vi "Main.vi"(8 "init information":string, 9 "model name":string, 11 "Module Admin":refnum<class "Delacor_lib_QMH_Cloneable Module Admin.lvclass">) -> ()   [LabVIEW 2022 SP3, in "Model Thread.lvlib"]
doc: "This template is based off of the Queued Message Handler design pattern and the Queued Message Handler project template that ships with LabVIEW.\n\nThe main difference is that the queue is private to this module and communication between modules is performed via Broadcast and Request events.\n\nRequest events are wrapped in public API methods and are handled in the Event Handling Loop (EHL) of this VI. Any module can register for Broadcast events sent by this module. The EHL generates messages based on user interface actions.\n\nThe Message Handling Loop (MHL) processes messages generated by the EHL, or by other messages. The messages are string values, so new messages can be added easily to the Message Cases case structure in the MHL. Each message cluster can also provide an optional value for Message Data, which is a variant that can be converted to whatever message-specific data is required.\n_____\nBased on DQMH Project Template 6.1.0.94."
uses:
  Model Thread.lvlib
  <vilib>/Delacor/Delacor QMH/Libraries/Cloneable Module Admin_class/Delacor_lib_QMH_Cloneable Module Admin.lvclass
  C:/Program Files (x86)/National Instruments/LabVIEW 2022/vi.lib/Delacor/Delacor QMH/Libraries/Module Admin_class/Delacor_lib_QMH_Module Admin.lvclass
  Abstract Model/Abstract Model.lvlibp/Abstract Model.lvclass
  Module Data--cluster.ctl
  <vilib>/Delacor/Delacor QMH/Libraries/Cloneable Module Admin_class/Delacor_lib_QMH_Cloneable Module Admin.lvclass/Delacor_lib_QMH_Cloneable Module Admin.ctl
  <vilib>/Delacor/Delacor QMH/Libraries/Message Queue_class/Delacor_lib_QMH_Message Queue.lvclass/Delacor_lib_QMH_Message Queue.ctl
  Stop Argument--cluster.ctl
  <vilib>/Delacor/Delacor QMH/Libraries/Module Admin_class/Delacor_lib_QMH_Module Admin.lvclass/Delacor_lib_QMH_Module Admin.ctl
  do action Argument--cluster.ctl
  <vilib>/Utility/miscctls.llb/LVPointTypeDef.ctl
  <vilib>/Delacor/Delacor QMH/Libraries/Cloneable Module Admin_class/Delacor_lib_QMH_Get Module ID.vi
  <vilib>/Delacor/Delacor QMH/Libraries/Message Queue_class/Delacor_lib_QMH_Enqueue Message (Single).vi
  <vilib>/Delacor/Delacor QMH/Libraries/Module Admin_class/Delacor_lib_QMH_Get External Launch.vi
  <vilib>/Utility/error.llb/Error Cluster From Error Code.vi
  <vilib>/ErrorRing/Error Ring.xnode
  <vilib>/Delacor/Delacor QMH/Libraries/Message Queue_class/Delacor_lib_QMH_Message Queue.lvclass
panel:
  in  "start query?":bool
  in  "Model copy":refnum<class "Abstract Model.lvclass">
  out "error out":errorcluster
  out "Status":string
  in  "Simulate EHL Error":bool
  in  "Simulate MHL Error":bool
  # "Other QMH Modules communicate with this Module via its Public API (wrappers for its Request Events).\n\nThis Module communicates with other Modules via its Broadcast Events.\nAny module that wants to get these messages, just registers for this module's Broadcast events."
  # "This template is for the Delacor Modified Queued Message Handler design pattern.\n\nSee the block diagram for more information on how to use this template."
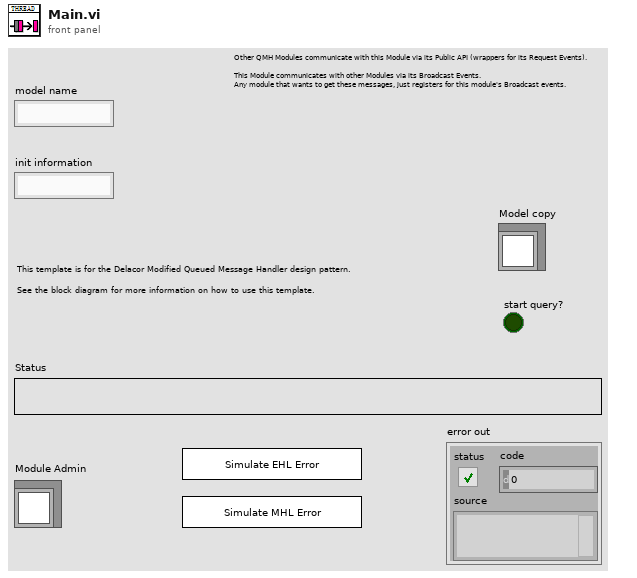
[diagram p1: front panel]
types:
  T1 = typedef "Model Thread.lvlib/Request Events--cluster.ctl" = cluster{"Stop Module":refnum<user-event>, "Show Panel":refnum<user-event>, "Hide Panel":refnum<user-event>, "Show Diagram":refnum<user-event>, "Get Module Execution Status":refnum<user-event>, "do action":refnum<user-event>}
  T2 = typedef "Model Thread.lvlib/Module Data--cluster.ctl" = cluster{"Status":string, "Model":refnum<class "Abstract Model.lvclass">}
  T3 = enum32{"invalid lock state", "Not Locked", "Locked (No Password)", "Password-protected"}
  T4 = typedef "Model Thread.lvlib/Stop Argument--cluster.ctl" = cluster{"Module ID":i32, "Origin":string, "Exit via Stop Module Req?":bool, "Wait for Module to stop?":bool}
  T5 = typedef "Model Thread.lvlib/do action Argument--cluster.ctl" = cluster{"Module ID":i32, "request":string}
  T6 = typedef "LVPointTypeDef.ctl" = cluster{"Horizontal":i16, "Vertical":i16}
  T7 = enum32{"Invalid", "Standard", "Closed", "Hidden", "Minimized", "Maximized"}
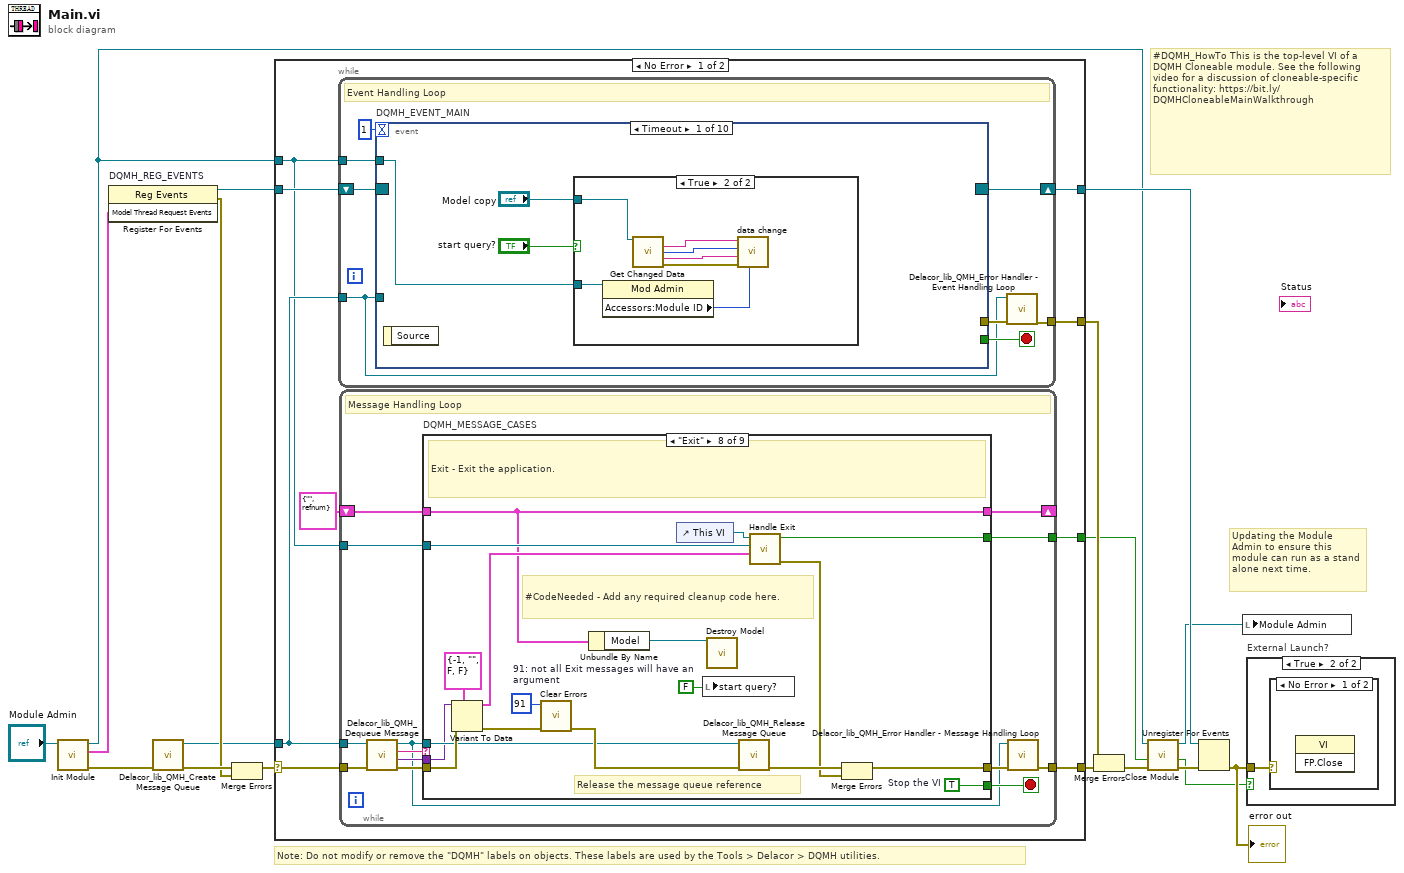
[diagram p0: block diagram]
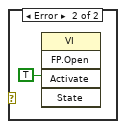
[diagram p3: hidden frame]
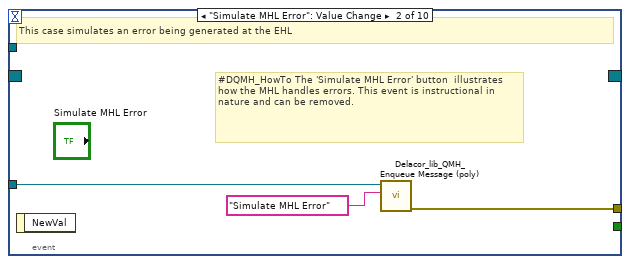
[diagram p5: hidden frame]
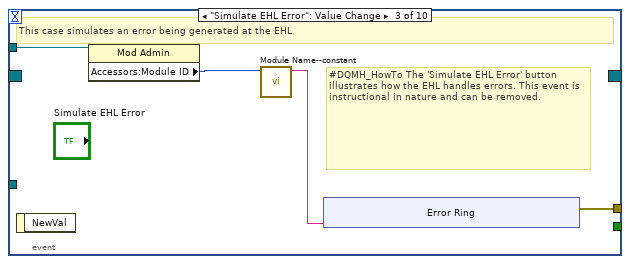
[diagram p6: hidden frame]
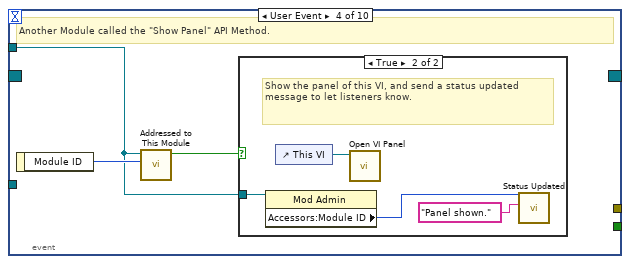
[diagram p7: hidden frame]
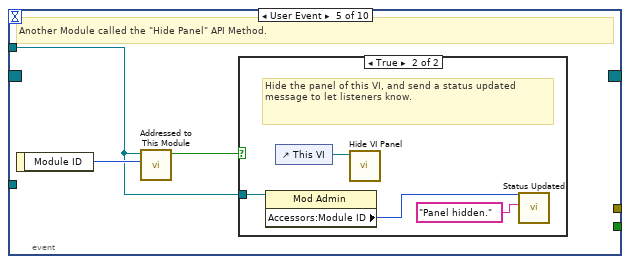
[diagram p9: hidden frame]
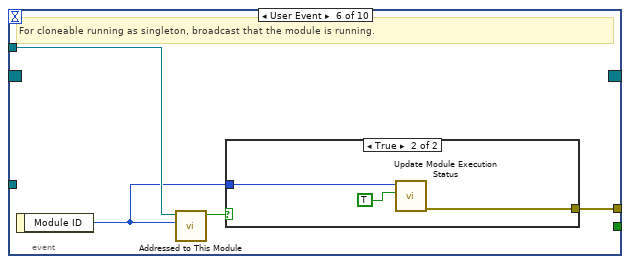
[diagram p11: hidden frame]
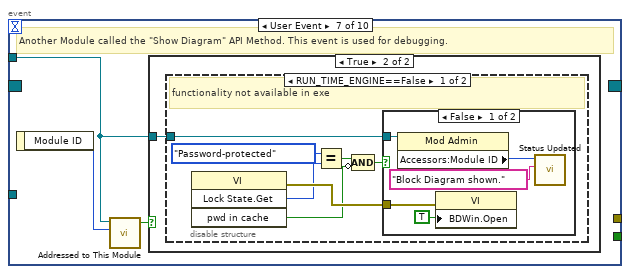
[diagram p13: hidden frame]
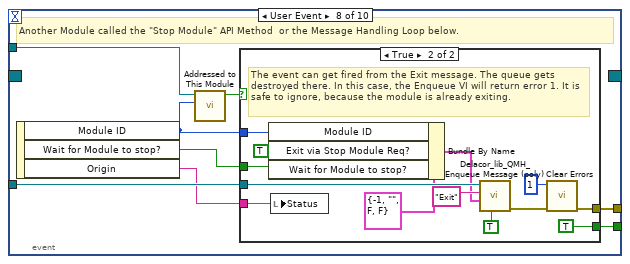
[diagram p17: hidden frame]
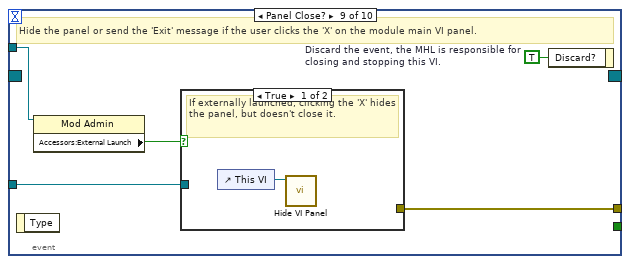
[diagram p19: hidden frame]
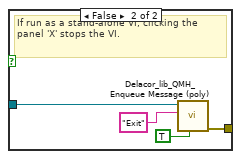
[diagram p20: hidden frame]
diagram:
  # "#DQMH_HowTo This is the top-level VI of a DQMH Cloneable module. See the following video for a discussion of cloneable-specific functionality: https://bit.ly/DQMHCloneableMainWalkthrough"
  # "Note: Do not modify or remove the \"DQMH\" labels on objects. These labels are used by the Tools > Delacor > DQMH utilities."
  # "Updating the Module Admin to ensure this module can run as a stand alone next time."
  n1 = call "Init Module.vi"("Cloneable Module Admin in"="Module Admin") -> ("error out"=w15:errorcluster, "Model Thread Request Events"=w7:T1, "Cloneable Module Admin out"=w4:refnum<class "Delacor_lib_QMH_Cloneable Module Admin.lvclass">)  [unwired: 8 in]
  n2 = register-events "DQMH_REG_EVENTS"(w7) -> (reference out=w8:refnum<event-registration>, error out=w10:errorcluster)  [unwired: 2 in]
  n3 = call <vilib>:"Delacor_lib_QMH_Create Message Queue.vi"("error in"=w15) -> ("error out"=w12:errorcluster, "Message Queue"=w6:refnum<class "Delacor_lib_QMH_Message Queue.lvclass">)  [unwired: 9 in]
  n4 = Merge Errors(w12, w10) -> (w11:errorcluster)
  n5 = case shown="No Error" w11 {
    selector: w11 -> [w25 w269]
    tunnel: [w27 w268] -> w16
    tunnel: [w24 w276] -> w9
    tunnel: w8 -> [w22 w276]
    tunnel: w6 -> [w21 w267]
    tunnel: [w26 _] -> w17
    tunnel: w4 -> [w20 w272]
    tunnel: [w19 _] -> w2
    frame No Error {
      n6 = while {
        tunnel: w21 -> [w29]
        shift-right: [w32] -> w24
        shift-left: w22 -> [w33]
        tunnel: [w34] -> w26
        tunnel: w20 -> [w30]
        stop <- w31 stop-if-true
        # "Event Handling Loop"
        n7 = event "DQMH_EVENT_MAIN" shown="[0] Timeout" {
          selector: w33 -> [_ _ _ _ _ _ _ _ _ _]
          dyn-events: [_ _ _ _ _ _ _ _ _ _] -> w32
          timeout: 1 -> [_ _ _ _ _ _ _ _ _ _]
          tunnel: [_ _ _ _ _ _ _ w100 _ _] -> w31
          tunnel: w29 -> [_ w47 _ _ _ _ _ w103 w119 w135]
          tunnel: [_ w48 w52 _ _ w77 _ w104 w122 w128] -> w35
          tunnel: w30 -> [w36 _ w51 w60 w67 w75 w81 w102 w120 w133]
          event Timeout {
            n8 = event-data() -> ()  [unwired: 1 in, 1 out]
            n9 = case shown="True" "start query?" {
              tunnel: "Model copy" -> [_ w45]
              tunnel: w36 -> [_ w40]
              frame False {
              }
              frame True {
                n10 = property class="Mod Admin"(reference=w40) -> ("Accessors:Module ID"=w39:i32)  [unwired: 1 in, 2 out]
                n11 = call-dynamic "Get Changed Data.vi"("Abstract Model in"=w45) -> ("view name"=w44:string, "view number"=w43:i32, "changed data"=w42:string, "error out"=w41:errorcluster)  [unwired: 10 in, 1 out]
                n12 = call "data change.vi"("Module ID"=w39, "error in"=w41, "changed data"=w42, "view number"=w43, "view name"=w44) -> ()  [unwired: 6 in, 1 out]
              }
            }
          }
          event "Simulate MHL Error": Value Change {
            # "#DQMH_HowTo The 'Simulate MHL Error' button  illustrates how the MHL handles errors. This event is instructional in nature and can be removed."
            # "This case simulates an error being generated at the EHL"
            n13 = event-data() -> ()  [unwired: 1 in, 1 out]
            n14 = call-poly <vilib>:"Delacor_lib_QMH_Enqueue Message (poly).vi"("Message"="Simulate MHL Error", "Message Queue in"=w47) -> ("error out"=w48:errorcluster)  [unwired: 8 in, 1 out]
          }
          event "Simulate EHL Error": Value Change {
            # "#DQMH_HowTo The 'Simulate EHL Error' button  illustrates how the EHL handles errors. This event is instructional in nature and can be removed."
            # "This case simulates an error being generated at the EHL"
            n15 = event-data() -> ()  [unwired: 1 in, 1 out]
            n16 = property class="Mod Admin"(reference=w51) -> ("Accessors:Module ID"=w50:i32)  [unwired: 1 in, 2 out]
            n17 = call "Module Name--constant.vi"("Module ID"=w50) -> ("Module Name"=w49:string)  [unwired: 10 in]
            n18 = xnode "Error Ring"("parameter 0"=w49) -> ("error out"=w52:errorcluster)
          }
          event User Event {
            # "Another Module called the \"Show Panel\" API Method."
            n19 = event-data() -> ("Module ID"=w61:i32)  [unwired: 1 in]
            n20 = call "Addressed to This Module.vi"("Module ID from Argument"=w61, "Module Admin"=w60) -> ("Addressed to this instance?"=w62:bool)  [unwired: 8 in, 1 out]
            n21 = case shown="True" w62 {
              tunnel: w60 -> [_ w64]
              frame False {
              }
              frame True {
                # "Show the panel of this VI, and send a status updated message to let listeners know."
                n22 = property class="Mod Admin"(reference=w64) -> ("Accessors:Module ID"=w63:i32)  [unwired: 1 in, 2 out]
                n23 = control-ref of="This VI"() -> (w66:refnum<vi>)
                n24 = call "Open VI Panel.vi"("VI"=w66) -> ()  [unwired: 10 in, 1 out]
                n25 = call "Status Updated.vi"("Status"="Panel shown." ("format string"), "Module ID"=w63) -> ()  [unwired: 9 in, 1 out]
              }
            }
          }
          event User Event {
            # "Another Module called the \"Hide Panel\" API Method."
            n26 = event-data() -> ("Module ID"=w68:i32)  [unwired: 1 in]
            n27 = call "Addressed to This Module.vi"("Module ID from Argument"=w68, "Module Admin"=w67) -> ("Addressed to this instance?"=w69:bool)  [unwired: 8 in, 1 out]
            n28 = case shown="True" w69 {
              tunnel: w67 -> [_ w71]
              frame False {
              }
              frame True {
                # "Hide the panel of this VI, and send a status updated message to let listeners know."
                n29 = property class="Mod Admin"(reference=w71) -> ("Accessors:Module ID"=w70:i32)  [unwired: 1 in, 2 out]
                n30 = control-ref of="This VI"() -> (w73:refnum<vi>)
                n31 = call "Hide VI Panel.vi"("VI"=w73) -> ()  [unwired: 10 in, 1 out]
                n32 = call "Status Updated.vi"("Status"="Panel hidden." ("format string"), "Module ID"=w70) -> ()  [unwired: 9 in, 1 out]
              }
            }
          }
          event User Event {
            # "For cloneable running as singleton, broadcast that the module is running."
            n33 = event-data() -> ("Module ID"=w74:i32)  [unwired: 1 in]
            n34 = call "Addressed to This Module.vi"("Module ID from Argument"=w74, "Module Admin"=w75) -> ("Addressed to this instance?"=w76:bool)  [unwired: 8 in, 1 out]
            n35 = case shown="True" w76 {
              tunnel: [_ w80] -> w77
              tunnel: w74 -> [_ w79]
              frame False {
              }
              frame True {
                n36 = call "Update Module Execution Status.vi"("Running?"=TRUE, "Module ID"=w79) -> ("error out"=w80:errorcluster)  [unwired: 9 in]
              }
            }
          }
          event User Event {
            # "Another Module called the \"Show Diagram\" API Method. This event is used for debugging."
            n37 = event-data() -> ("Module ID"=w82:i32)  [unwired: 1 in]
            n38 = call "Addressed to This Module.vi"("Module ID from Argument"=w82, "Module Admin"=w81) -> ("Addressed to this instance?"=w83:bool)  [unwired: 8 in, 1 out]
            n39 = case shown="True" w83 {
              tunnel: w81 -> [_ w84]
              frame False {
              }
              frame True {
                n40 = disable-structure shown="RUN_TIME_ENGINE==False" {
                  disable-tunnel: w84 -> [w85 _]
                  frame condition #0 (active) {
                    # "functionality not available in exe"
                    n41 = invoke class="VI" method="Lock State.Get"() -> (error out=w91:errorcluster, "Get Lock State"=w90:T3, "pwd in cache"=w87:bool)  [unwired: 4 in, 1 out]
                    n42 = Equal?(x=T3."Password-protected", y=w90) -> (x = y?=w88:bool)
                    n43 = Compound Arithmetic op=AND(w88, invert w87) -> (w86:bool)
                    n44 = case shown="False" w86 {
                      tunnel: w91 -> [w96 _]
                      tunnel: w85 -> [w93 _]
                      frame False {
                        n45 = property class="Mod Admin"(reference=w93) -> ("Accessors:Module ID"=w92:i32)  [unwired: 1 in, 2 out]
                        n46 = property class="VI"(error in=w96, "BDWin.Open"=TRUE ("Block Diagram Window:Open")) -> ()  [unwired: 1 in, 2 out]
                        n47 = call "Status Updated.vi"("Status"="Block Diagram shown." ("format string"), "Module ID"=w92) -> ()  [unwired: 9 in, 1 out]
                      }
                      frame True {
                        # "Password-protected VI, and the password is not in the cache. Do not show the diagram."
                      }
                    }
                  }
                  frame condition #1 {
                  }
                }
              }
            }
          }
          event User Event {
            # "Another Module called the \"Stop Module\" API Method  or the Message Handling Loop below."
            n48 = event-data() -> ("Module ID"=w98:i32, "Wait for Module to stop?"=w99:bool, "Origin"=w97:string)  [unwired: 1 in]
            n49 = call "Addressed to This Module.vi"("Module ID from Argument"=w98, "Module Admin"=w102) -> ("Addressed to this instance?"=w101:bool)  [unwired: 8 in, 1 out]
            n50 = case shown="True" w101 {
              tunnel: [_ w116] -> w104
              tunnel: w103 -> [_ w112]
              tunnel: [_ TRUE] -> w100
              tunnel: w99 -> [_ w107]
              tunnel: w98 -> [_ w109]
              tunnel: w97 -> [_ w105]
              frame False {
              }
              frame True {
                # "The event can get fired from the Exit message. The queue gets destroyed there. In this case, the Enqueue VI will return error 1. It is safe to ignore, because the module is already exiting."
                n51 = Bundle By Name(cluster=T4 {"Module ID"=-1, "Origin"="", "Exit via Stop Module Req?"=FALSE, "Wait for Module to stop?"=FALSE} ("Stop Argument"), "Module ID"=w109, "Exit via Stop Module Req?"=TRUE, "Wait for Module to stop?"=w107) -> (w106:T4)
                n52 = local write "Status"(w105) -> ()
                n53 = call-poly <vilib>:"Delacor_lib_QMH_Enqueue Message (poly).vi"("Priority Message? (F)"=TRUE, "Message Data"=w106, "Message"="Exit", "Message Queue in"=w112) -> ("error out"=w117:errorcluster)  [unwired: 6 in, 1 out]
                n54 = call <vilib>:"Clear Errors.vi"("error in (no error)"=w117, "specific error code to clear (0: all)"=1) -> ("error out"=w116:errorcluster)  [unwired: 4 in, 1 out]
              }
            }
          }
          event Panel Close? {
            w121 = TRUE  # Discard the event, the MHL is responsible for closing and stopping this VI.
            # "Hide the panel or send the 'Exit' message if the user clicks the 'X' on the module main VI panel."
            n55 = event-data() -> ()  [unwired: 1 in, 1 out]
            n56 = property class="Mod Admin"(reference=w120) -> ("Accessors:External Launch"=w118:bool)  [unwired: 1 in, 2 out]
            n57 = case shown="True" w118 {
              tunnel: w119 -> [_ w126]
              tunnel: [_ w127] -> w122
              frame True {
                # "If externally launched, clicking the 'X' hides the panel, but doesn't close it."
                n58 = control-ref of="This VI"() -> (w123:refnum<vi>)
                n59 = call "Hide VI Panel.vi"("VI"=w123) -> ()  [unwired: 10 in, 1 out]
              }
              frame False {
                # "If run as a stand-alone VI, clicking the panel 'X' stops the VI."
                n60 = call-poly <vilib>:"Delacor_lib_QMH_Enqueue Message (poly).vi"("Priority Message? (F)"=TRUE, "Message"="Exit", "Message Queue in"=w126) -> ("error out"=w127:errorcluster)  [unwired: 7 in, 1 out]
              }
            }
            n61 = event-data("Discard?"=w121) -> ()  [unwired: 1 in, 1 out]
          }
          event User Event {
            # "Another Module called the \"do action\" API Method."
            n62 = event-data() -> ("Module ID"=w130:i32, "request"=w129:string)  [unwired: 1 in]
            n63 = Bundle(cluster=T5 {"Module ID"=-1, "request"=""} ("do action Argument"), "Module ID"=w130, "request"=w129) -> (w131:T5)
            n64 = call "Addressed to This Module.vi"("Module ID from Argument"=w130, "Module Admin"=w133) -> ("Addressed to this instance?"=w134:bool)  [unwired: 8 in, 1 out]
            n65 = case shown="True" w134 {
              tunnel: w135 -> [_ w139]
              tunnel: w131 -> [_ w137]
              tunnel: [_ w136] -> w128
              frame False {
              }
              frame True {
                n66 = call-poly <vilib>:"Delacor_lib_QMH_Enqueue Message (poly).vi"("Message Data"=w137, "Message"="do action", "Message Queue in"=w139) -> ("error out"=w136:errorcluster)  [unwired: 7 in, 1 out]
              }
            }
          }
        }
        n67 = call-dynamic "Delacor_lib_QMH_Error Handler - Event Handling Loop.vi"("error in"=w35, "Message Queue in"=w29) -> ("dup error in"=w34:errorcluster)  [unwired: 8 in, 1 out]
      }
      n68 = while {
        tunnel: w21 -> [w143]
        shift-right: [w147] -> _
        shift-left: T2 {"Status"="", "Model"=refnum} ("Data Cluster") -> [w148]
        tunnel: w25 -> [w151]
        tunnel: [w149] -> w27
        tunnel: w20 -> [w141]
        tunnel: [w140] -> w19
        stop <- w146 stop-if-true
        # "Message Handling Loop"
        n69 = call-dynamic "Delacor_lib_QMH_Dequeue Message.vi"("error in"=w151, "Message Queue in"=w143) -> ("error out"=w150:errorcluster, "Message Data"=w144:variant, "Message"=w145:string, "Message Queue out"=w142:refnum<class "Delacor_lib_QMH_Message Queue.lvclass">)  [unwired: 6 in]
        n70 = case "DQMH_MESSAGE_CASES" shown="\"Exit\"" w145 {
          selector: w145 -> [_ _ _ _ _ _ _ _ w254]
          tunnel: w142 -> [_ _ _ _ _ w203 _ w244 _]
          tunnel: w150 -> [w177 w184 w196 w199 w201 w212 w225 w250 w256]
          tunnel: [w175 w184 w186 w198 w201 w208 w224 w247 w257] -> w152
          tunnel: w148 -> [w168 w183 w193 w197 w200 w207 w222 w235 w255]
          tunnel: [w167 w183 w192 w197 w200 w207 w222 w235 w255] -> w147
          tunnel: [_ _ _ _ _ _ _ w243 _] -> w146
          tunnel: w144 -> [_ _ w185 _ _ w206 _ w241 _]
          tunnel: w141 -> [w163 _ w189 _ _ w205 w220 w237 w252]
          tunnel: [_ _ _ _ _ _ _ w239 _] -> w140
          frame "Initialize" {
            # "Initialize - Any operation that needs to be done before the module can receive messages. Synchronize Caller Events.vi will inform Start Module.vi that the module has launched and is ready to receive messages. Module Did Init.vi will broadcast that the module initialized."
            n71 = call "Synchronize Caller Events.vi"("error in (no error)"=w177, "Module Admin"=w163) -> ("error out"=w176:errorcluster, "Module Admin out"=w162:refnum<class "Delacor_lib_QMH_Cloneable Module Admin.lvclass">)  [unwired: 8 in]
            n72 = property class="Mod Admin"(reference=w162) -> ("Accessors:Module ID"=w160:i32, "Accessors:External Launch"=w164:bool)  [unwired: 1 in, 2 out]
            n73 = call "load model plugin.vi"("model name"="model name") -> ("Model plugin"=w158:refnum<class "Abstract Model.lvclass">, "error out"=w159:errorcluster)  [unwired: 13 in]
            n74 = call-dynamic "Obtain Model.vi"("Abstract Model in"=w158, "init information"="init information", "error in (no error)"=w159) -> ("Abstract Model out"=w154:refnum<class "Abstract Model.lvclass">, "error out"=w155:errorcluster)  [unwired: 11 in]
            n75 = flat-sequence {
              tunnel: w155 -> [w181]
              tunnel: w154 -> [w182]
              tunnel: [w182] -> w153
              frame #0 {
                n76 = Not(x=w181) -> (.not. x?=w180:bool)
                n77 = local write "Model copy"(w182) -> ()
                n78 = local write "start query?"(w180) -> ()
              }
            }
            n79 = call "Module Name--constant.vi"("Module ID"=w160) -> ("Module Name"=w172:string)  [unwired: 10 in]
            n80 = property class="VI"("Front Panel.Title"=w172) -> (reference out=w174:refnum<vi>, error out=w179:errorcluster)  [unwired: 2 in]
            n81 = Select(t=T7."Hidden" ("State"), s=w164, f=T7."Standard" ("State")) -> (s? t:f=w169:T7)
            n82 = invoke class="VI" method="FP.Open"(reference=w174, error in=w179, "State"=w169) -> (reference out=w173:refnum<vi>, error out=w178:errorcluster)  [unwired: 2 in, 3 out]
            n83 = call "Module Name--constant.vi"("Module ID"=w160) -> ("Module Name"=w165:string)  [unwired: 10 in]
            n84 = Bundle By Name(cluster=w168, "Model"=w153) -> (w167:T2)
            n85 = invoke class="VI" method="FP.Center"(reference=w173, error in=w178) -> ()  [unwired: 1 in, 3 out]
            n86 = property on="Pane" class="Pane"("Origin"=T6 {"Horizontal"=0, "Vertical"=0}) -> ()  [unwired: 2 in, 2 out]
            n87 = call "Module Did Init.vi"("error in (no error)"=w176, "Initialized?"=TRUE, "Origin"=w165, "Module ID"=w160) -> ("error out"=w175:errorcluster)  [unwired: 7 in]
          }
          frame "---Module Specific---" {
            # "Separator -- The following cases handle messages specific to this Module."
          }
          frame "do action" {
            n88 = property class="Mod Admin" props=["Accessors:Module ID"](reference=w189) -> ()  [unwired: 1 in, 3 out]
            n89 = Unbundle By Name(w193) -> ("Model"=w188:refnum<class "Abstract Model.lvclass">)
            n90 = Variant To Data(error in=w196, type=T5 {"Module ID"=-1, "request"=""} ("do action Argument"), Variant=w185) -> (data=w194:T5, error out=w186:errorcluster)
            n91 = Unbundle By Name(w194) -> ("request"=w191:string)
            n92 = call-dynamic "Do Action.vi"("Abstract Model in"=w188, "request"=w191) -> ("Abstract Model out"=w190:refnum<class "Abstract Model.lvclass">, "error out"=w187:errorcluster)  [unwired: 12 in]
            n93 = Not(x=w187) -> ()  [unwired: 1 out]
            n94 = Bundle By Name(cluster=w193, "Model"=w190) -> (w192:T2)
          }
          frame "---Copy This Frame---" {
            # "Duplicate this frame when creating new messages.  Change this comment in the duplicated frame to describe this message."
            n95 = Merge Errors(w199) -> (w198:errorcluster)
          }
          frame "---Exit and Error Handling---" {
            # "Separator - the following cases handle errors and exit messages."
          }
          frame "Error" {
            # "#CodeRecommended - If you ever change the name of this \"Error\" message, you'll need to update the name in the Check Loop Error.vi as well."
            # "#CodeRecommended - If the module is running in standalone mode (External Launch = FALSE), this code will pop up an error dialog and call the 'Exit' message if an error occurs. Add more fine-grained error handling here."
            # "Error - Check the error message data and respond accordingly. This message is sent by the \"Error Handler\" VIs at the end of each loop in this application."
            n96 = property class="Mod Admin"(reference=w205) -> ("Accessors:External Launch"=w204:bool, "Accessors:Module ID"=w202:i32)  [unwired: 1 in, 2 out]
            n97 = Variant To Data(error in=w212, type=errorcluster {"status"=FALSE, "code"=0, "source"=""} ("error constant"), Variant=w206) -> (data=w213:errorcluster, error out=w210:errorcluster)
            n98 = call "Error Reported.vi"("Error"=w213, "Module ID"=w202) -> ()  [unwired: 9 in, 1 out]
            n99 = case shown="False" w204 {
              tunnel: [w218 _] -> w209
              tunnel: w203 -> [w216 _]
              tunnel: w213 -> [w217 _]
              frame False {
                # "If the module is running standalone, then pop up an error dialog and call the \"Exit\" message."
                n100 = call <vilib>:"Simple Error Handler.vi"("error in (no error)"=w217) -> ()  [unwired: 4 in, 5 out]
                n101 = call-poly <vilib>:"Delacor_lib_QMH_Enqueue Message (poly).vi"("Priority Message? (F)"=TRUE, "Message"="Exit", "Message Queue in"=w216) -> ("error out"=w218:errorcluster)  [unwired: 7 in, 1 out]
              }
              frame True {
                # "If the module was launched externally, calling the Error Reported broadcast VI is the only action performed by the \"Error\" message. The module's caller can then process the error appropriately."
              }
            }
            n102 = Merge Errors(w210, w209) -> (w208:errorcluster)
            n103 = local write "error out"(w208) -> ()
          }
          frame "Simulate MHL Error" {
            # "#DQMH_HowTo The 'Simulate MHL Error' button  illustrates how the MHL handles errors. This event is instructional in nature and can be removed."
            # "Simulate an error occurring at the MHL"
            n104 = property class="Mod Admin"(reference=w220) -> ("Accessors:Module ID"=w221:i32)  [unwired: 1 in, 2 out]
            n105 = call "Module Name--constant.vi"("Module ID"=w221) -> ("Module Name"=w219:string)  [unwired: 10 in]
            n106 = xnode "Error Ring"("parameter 0"=w219) -> ("error out"=w223:errorcluster)
            n107 = Merge Errors(w225, w223) -> (w224:errorcluster)
          }
          frame "Exit" {
            w242 = 91  # 91: not all Exit messages will have an argument
            w243 = TRUE  # Stop the VI
            # "#CodeNeeded - Add any required cleanup code here."
            # "Release the message queue reference"
            # "Exit - Exit the application."
            n108 = Variant To Data(error in=w250, type=T4 {"Module ID"=-1, "Origin"="", "Exit via Stop Module Req?"=FALSE, "Wait for Module to stop?"=FALSE} ("Stop Argument"), Variant=w241) -> (data=w238:T4, error out=w245:errorcluster)
            n109 = call <vilib>:"Clear Errors.vi"("error in (no error)"=w245, "specific error code to clear (0: all)"=w242) -> ("error out"=w249:errorcluster)  [unwired: 4 in, 1 out]
            n110 = Unbundle By Name(w235) -> ("Model"=w234:refnum<class "Abstract Model.lvclass">)
            n111 = control-ref of="This VI"() -> (w236:refnum<vi>)
            n112 = local write "start query?"(FALSE ("start query?")) -> ()
            n113 = call-dynamic "Destroy Model.vi"("Abstract Model in"=w234) -> ()  [unwired: 13 in, 2 out]
            n114 = call-dynamic "Delacor_lib_QMH_Release Message Queue.vi"("error in"=w249, "Message Queue"=w244) -> ("error out"=w248:errorcluster)  [unwired: 9 in]
            n115 = call "Handle Exit.vi"("Stop Argument"=w238, "Module Admin in"=w237, "VI reference"=w236) -> ("error out"=w246:errorcluster, "Wait for Stop?"=w239:bool)  [unwired: 7 in]
            n116 = Merge Errors(w248, w246) -> (w247:errorcluster)
          }
          frame Default {
            # "'Default' case only runs if there is a message that isn't defined in any of the other cases.  Output a programming error."
            n117 = property class="Mod Admin"(reference=w252) -> ("Accessors:Module ID"=w251:i32)  [unwired: 1 in, 2 out]
            n118 = call "Module Name--constant.vi"("Module ID"=w251) -> ("Module Name"=w253:string)  [unwired: 10 in]
            n119 = xnode "Error Ring"("parameter 0"=w254, "parameter 1"=w253) -> ("error out"=w258:errorcluster)
            n120 = Merge Errors(w256, w258) -> (w257:errorcluster)
          }
        }
        n121 = call-dynamic "Delacor_lib_QMH_Error Handler - Message Handling Loop.vi"("error in"=w152, "Message Queue in"=w142) -> ("dup error in"=w149:errorcluster)  [unwired: 8 in, 1 out]
      }
    }
    frame Error {
      n122 = call "Synchronize Caller Events.vi"("Module Admin"=w272) -> ("Module Admin out"=w271:refnum<class "Delacor_lib_QMH_Cloneable Module Admin.lvclass">)  [unwired: 9 in, 1 out]
      n123 = property class="Mod Admin"(reference=w271) -> ("Accessors:Module ID"=w270:i32)  [unwired: 1 in, 2 out]
      n124 = call-dynamic "Delacor_lib_QMH_Release Message Queue.vi"("error in"=w269, "Message Queue"=w267) -> ("error out"=w268:errorcluster)  [unwired: 9 in]
      n125 = call "Module Name--constant.vi"("Module ID"=w270) -> ("Module Name"=w275:string)  [unwired: 10 in]
      n126 = Format Into String(format string="An error occurred during initialization. %s is no longer running.", w275) -> (resulting string=w273:string)  [unwired: 2 in, 1 out]
      n127 = call "Error Reported.vi"("Additional Information"=w273, "Error"=w268, "Module ID"=w270) -> ()  [unwired: 8 in, 1 out]
    }
  }
  n128 = Merge Errors(w17, w16) -> (w18:errorcluster)
  n129 = call "Close Module.vi"("error in"=w18, "Wait for stop?"=w2, "Module Admin in"=w4) -> ("error out"=w14:errorcluster, "External Launch"=w1:bool, "Module Admin out"=w3:refnum<class "Delacor_lib_QMH_Cloneable Module Admin.lvclass">)  [unwired: 6 in]
  n130 = Unregister For Events(event registration refnum=w9, error in=w14) -> (error out=w13:errorcluster)
  "error out" <- w13
  n131 = local write "Module Admin"(w3) -> ()
  n132 = case "External Launch?" shown="True" w1 {
    tunnel: w13 -> [_ w277]
    frame False {
    }
    frame True {
      n133 = case shown="No Error" w277 {
        frame No Error {
          n134 = invoke class="VI" method="FP.Close"() -> ()  [unwired: 3 in, 3 out]
        }
        frame Error {
          n135 = invoke class="VI" method="FP.Open"("Activate"=TRUE ("Activate?")) -> ()  [unwired: 4 in, 5 out]
        }
      }
    }
  }
